vi "FRCts20_Backend_EventRoot_GET_reform.vi"(8 "error in (no error)":errorcluster, 11 "recordset data":variant[][](array[variant])) -> (0 "error out":errorcluster, 3 "data string":string)   [LabVIEW 2014, in "FRCts20_Backend_Engine.lvlib"]
doc: "Parses and returns all the events' data"
uses:
  FRCts20_Backend_Engine.lvlib
  FRCts20_Backend_API/FRCts20_Backend_API_EventRoot.ctl
  FRCts20_Backend_DBCluster_EventRoot_GET.ctl
  <vilib>/addons/database/_DB Variant To Data/Database Variant To Data.xnode
  FRCts20_Backend_API/FRCts20_Backend_API.lvlib
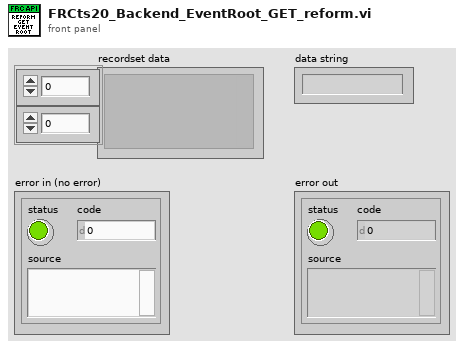
[diagram p1: front panel]
types:
  T1 = typedef "FRCts20_Backend_API.lvlib/FRCts20_Backend_API_EventRoot.ctl" = cluster{"Event":cluster{"Event Index":u32, "EventID":u32, "EventSubtype":string, "EventSubtypeID":u32, "DistrictCode":string, "DistrictID":u32, "Event Name":string, "Venue":string, "City":string, "StateProvince":string, "Country":string, "Start Time":timestamp, "End Time":timestamp, "Year":u32, "NumberOfTeams":u32, "URLTeamlist":string, "EventCode":string, "OpenIssues":u8, "IsLive":bool}[], "APIReturn":string}
  T2 = typedef "FRCts20_Backend_Engine.lvlib/FRCts20_Backend_DBCluster_EventRoot_GET.ctl" = cluster{"EventIndex":u32, "EventName":string, "StartTime":timestamp, "EndTime":timestamp, "OpenIssues":u8, "IsLive":u8}
  T3 = cluster{"Event Index":u32, "EventID":u32, "EventSubtype":string, "EventSubtypeID":u32, "DistrictCode":string, "DistrictID":u32, "Event Name":string, "Venue":string, "City":string, "StateProvince":string, "Country":string, "Start Time":timestamp, "End Time":timestamp, "Year":u32, "NumberOfTeams":u32, "URLTeamlist":string, "EventCode":string, "OpenIssues":u8, "IsLive":bool}[]
  T4 = cluster{"Event Index":u32, "EventID":u32, "EventSubtype":string, "EventSubtypeID":u32, "DistrictCode":string, "DistrictID":u32, "Event Name":string, "Venue":string, "City":string, "StateProvince":string, "Country":string, "Start Time":timestamp, "End Time":timestamp, "Year":u32, "NumberOfTeams":u32, "URLTeamlist":string, "EventCode":string, "OpenIssues":u8, "IsLive":bool}
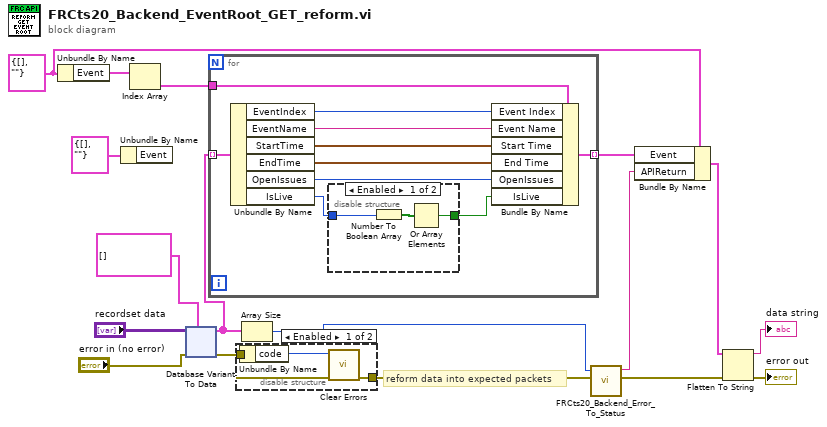
[diagram p0: block diagram]
diagram:
  w9 = T1 {"Event"=[], "APIReturn"=""} ("Competitions")
  # "reform data into expected packets"
  n1 = Unbundle By Name(w9) -> ("Event"=w7:T3)
  n2 = Unbundle By Name(T1 {"Event"=[], "APIReturn"=""} ("Events")) -> ()  [unwired: 1 out]
  n3 = Index Array(array=w7) -> (element=w6:T4)  [unwired: 1 in]
  n4 = xnode "Database Variant To Data"("database variant"="recordset data", "error in (no error)"="error in (no error)", "type"=T2[] []) -> ("data"=w1:T2[], "error out"=w3:errorcluster)
  n5 = for {
    tunnel: w1 -> [w27] mode=indexing
    tunnel: w6 -> [w26]
    tunnel: [w24] -> w8 mode=indexing
    n6 = Unbundle By Name(w27) -> ("EventIndex"=w23:u32, "EventName"=w25:string, "StartTime"=w22:timestamp, "EndTime"=w21:timestamp, "OpenIssues"=w20:u8, "IsLive"=w18:u8)
    n7 = disable-structure shown="Enabled" {
      disable-tunnel: [w29 w31] -> w19
      disable-tunnel: w18 -> [w28 w31]
      frame Enabled {
        n8 = Number To Boolean Array(number=w28) -> (Boolean array=w30:bool[])
        n9 = Or Array Elements(Boolean array=w30) -> (logical OR=w29:bool)
      }
      frame Disabled {
      }
    }
    n10 = Bundle By Name(cluster=w26, "Event Index"=w23, "Event Name"=w25, "Start Time"=w22, "End Time"=w21, "OpenIssues"=w20, "IsLive"=w19) -> (w24:T4)
  }
  n11 = disable-structure shown="Enabled" {
    disable-tunnel: w3 -> [w33 w35]
    disable-tunnel: [w32 w35] -> w2
    frame Enabled {
      n12 = Unbundle By Name(w33) -> ("code"=w34:i32)
      n13 = call <vilib>:"Clear Errors.vi"("error in (no error)"=w33, "specific error code to clear (0: all)"=w34) -> ("error out"=w32:errorcluster)  [unwired: 4 in, 1 out]
    }
    frame Disabled {
    }
  }
  n14 = Array Size(array=w1) -> (size(s)=w12:i32)
  n15 = call "FRCts20_Backend_Error_To_Status.vi"("error in (no error)"=w2, "rows affected"=w12) -> ("error out"=w13:errorcluster, "String"=w14:string)  [unwired: 8 in]
  n16 = Bundle By Name(cluster=w9, "Event"=w8, "APIReturn"=w14) -> (w15:T1)
  n17 = Flatten To String(anything=w15, error in (no error)=w13) -> (data string=→"data string":string, error out=→"error out":errorcluster)  [unwired: 2 in, 1 out]
